vi "Calculation_test.vi"() -> (0 "New Values In":string[][](array[string])=[["Test data5"]], 1 "New Chs In":string[](array[string])=["30-10-03:New:Channel new5"])   [LabVIEW 2010]
uses:
  Results_plotter_Global.vi
panel:
  in  "New Chs In 2":string[](array[string])=["30-10-03:New:Channel new5"]
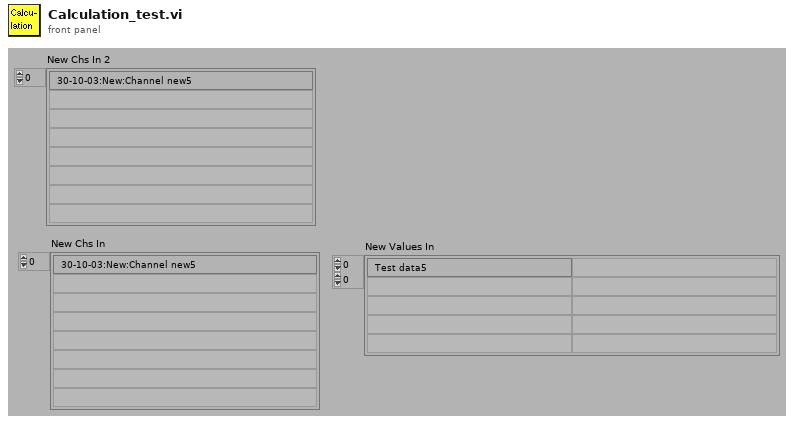
[diagram p1: front panel]
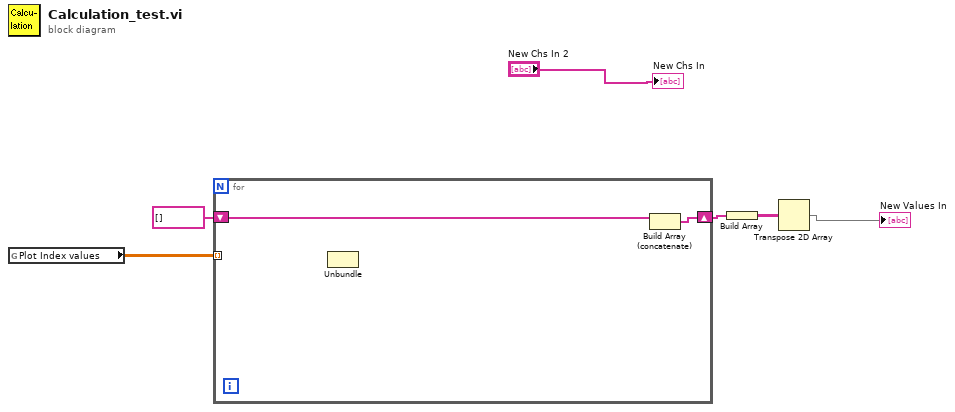
[diagram p0: block diagram]
diagram:
  n1 = global read "Results_plotter_Global.vi" "Plot Index values"() -> (w6:dbl[][])
  n2 = for {
    tunnel: w6 -> [_] mode=indexing
    shift-right: [w8] -> w4
    shift-left: string[] [] -> [w7]
    n3 = Unbundle() -> ()  [unwired: 1 in, 2 out]
    n4 = Build Array (concatenate)(w7) -> (w8:string[])  [unwired: 1 in]
  }
  n5 = Build Array(w4) -> (w3:string[][])
  n6 = Transpose 2D Array(2D array=w3) -> (transposed array=→"New Values In":string[][])
  "New Chs In" <- "New Chs In 2"
